vi "PXI-Set AO Value.vi"(0 "physical channel":tag, 7 "Value":dbl, 11 "error in":errorcluster) -> (15 "error out":errorcluster)   [LabVIEW 2020]
uses:
  <vilib>/DAQmx/write.llb/DAQmx Write (Analog 1D DBL 1Chan NSamp).vi
  <vilib>/DAQmx/create/channels.llb/DAQmx Create Channel (AO-Voltage-Basic).vi
  <vilib>/DAQmx/configure/timing.llb/DAQmx Timing (Sample Clock).vi
  <vilib>/DAQmx/miscellaneous.llb/DAQmx Fill In Error Info.vi
  <resource>/objmgr/daqmx.rc
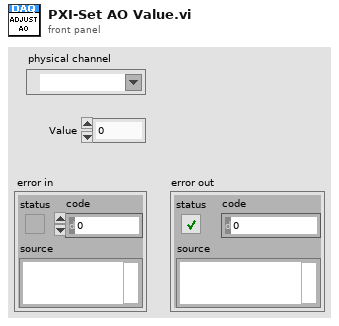
[diagram p1: front panel]
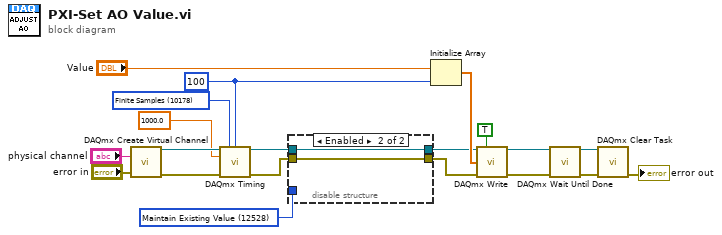
[diagram p0: block diagram]
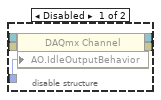
[diagram p2: hidden frame]
diagram:
  w7 = 12528 items=["Zero Volts"=12526, "High-Impedance"=12527, "Maintain Existing Value"=12528] ("AO.IdleOutputBehavior")
  w11 = 100 ("samples per channel")
  w12 = 10178 items=["Finite Samples"=10178, "Continuous Samples"=10123, "Hardware Timed Single Point"=12522] ("sample mode")
  n1 = call-poly <vilib>:"DAQmx Create Virtual Channel.vi"("physical channels"="physical channel", "error in"="error in") -> ("task out"=w20:refnum<k21>, "error out"=w19:errorcluster)  [unwired: 12 in]
  n2 = call-poly <vilib>:"DAQmx Timing.vi"("task/channels in"=w20, "sample mode"=w12, "samples per channel"=w11, "rate"=1000.0, "error in"=w19) -> ("task out"=w8:refnum<k21>, "error out"=w3:errorcluster)  [unwired: 9 in]
  n3 = disable-structure shown="Enabled" {
    disable-tunnel: w8 -> [w25 w27]
    disable-tunnel: w7 -> [w24 _]
    disable-tunnel: [w23 w27] -> w6
    disable-tunnel: w3 -> [w22 w26]
    disable-tunnel: [w21 w26] -> w2
    frame Disabled {
      n4 = property class="DAQmx Channel"(reference=w25, error in=w22, "AO.IdleOutputBehavior"=w24) -> (reference out=w23:refnum<k21>, error out=w21:errorcluster)
    }
    frame Enabled {
    }
  }
  n5 = Initialize Array("Value", w11) -> (w9:dbl[])
  n6 = call-poly <vilib>:"DAQmx Write.vi"("task/channels in"=w6, "auto start"=TRUE, "data"=w9, "error in"=w2) -> ("task out"=w14:refnum<k21>, "error out"=w15:errorcluster)  [unwired: 9 in, 1 out]
  n7 = call <vilib>:"DAQmx Wait Until Done.vi"("task/channels in"=w14, "error in"=w15) -> ("task out"=w16:refnum<k21>, "error out"=w17:errorcluster)  [unwired: 12 in]
  n8 = call <vilib>:"DAQmx Clear Task.vi"("task in"=w16, "error in"=w17) -> ("error out"=→"error out":errorcluster)  [unwired: 13 in]
